vi "coerce_demux_command.vi"(1 "U8 code":u8) -> (0 "Demux command":T1)   [LabVIEW 2012]
uses:
  Common/demux_command.ctl
panel:
  # "Coerce a U8 into an \"I2C command\" enum."
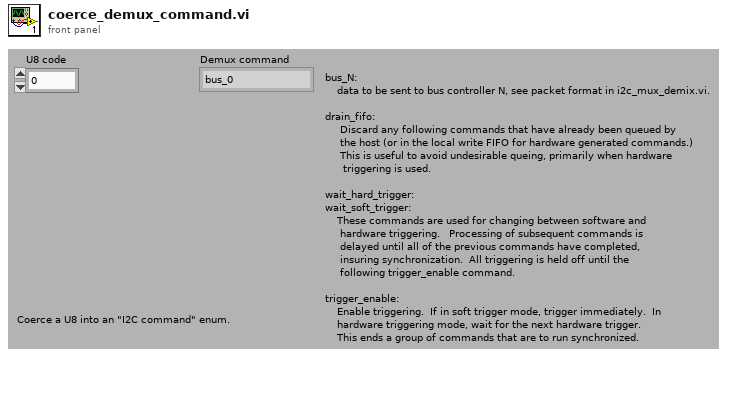
[diagram p1: front panel]
types:
  T1 = typedef "demux_command.ctl" = enum8{"bus_0", "bus_1", "bus_2", "invalid_3", "invalid_4", "drain_fifo", "wait_hard_trigger", "wait_soft_trigger", "trigger_enable"}
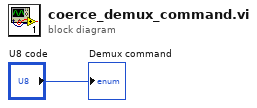
[diagram p0: block diagram]
diagram:
  "Demux command" <- "U8 code"
